vi "CMI ckd2 Set Divider Factor.vi"(8 "error in":errorcluster, 10 "division factor (1)":i32=1, 11 "session":T1) -> (0 "error out":errorcluster, 3 "session out":T1)   [LabVIEW 2020, in "AWG.lvlib"]
doc: "Sets division factor to main channel."
uses:
  AWG.lvlib
  CMI ckd2 Session.ctl
  CMI ckd2 Source Mode.ctl
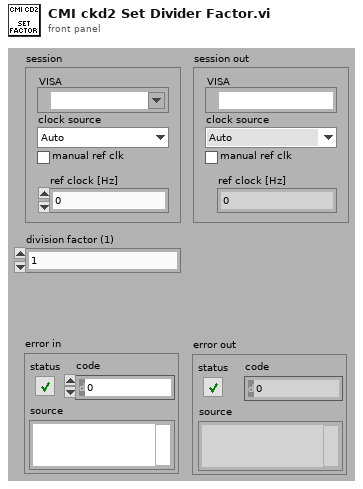
[diagram p1: front panel]
types:
  T1 = typedef "AWG.lvlib/CMI ckd2 Session.ctl" = cluster{"VISA":refnum<visa-resource-name>, "clock source":T2, "manual ref clk":bool, "ref clock [Hz]":dbl}
  T2 = typedef "AWG.lvlib/CMI ckd2 Source Mode.ctl" = enum16{"Auto", "LF clock", "HF clock", "Internal"}
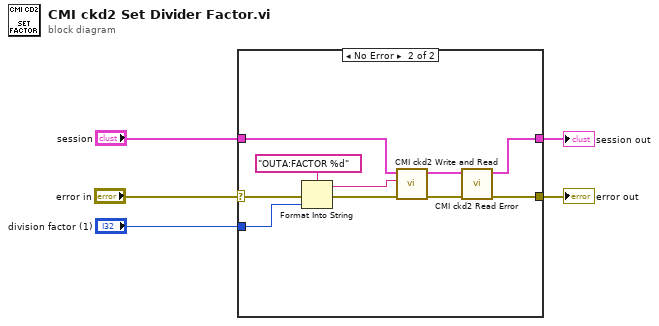
[diagram p0: block diagram]
diagram:
  n1 = case shown="No Error" "error in" {
    selector: "error in" -> [w6 w16]
    tunnel: [w7 w9] -> w3
    tunnel: [w6 w8] -> w5
    tunnel: "session" -> [w7 w17]
    tunnel: "division factor (1)" -> [_ w12]
    frame Error {
    }
    frame No Error {
      n2 = Format Into String(format string="OUTA:FACTOR %d", error in=w16, w12) -> (resulting string=w14:string, error out=w13:errorcluster)  [unwired: 1 in]
      n3 = call "CMI ckd2 Write and Read.vi"("error in"=w13, "command"=w14, "session"=w17) -> ("error out"=w11:errorcluster, "session out"=w10:T1)  [unwired: 6 in, 1 out]
      n4 = call "CMI ckd2 Read Error.vi"("error in"=w11, "session"=w10) -> ("error out"=w8:errorcluster, "session out"=w9:T1)  [unwired: 7 in, 1 out]
    }
  }
  "error out" <- w5
  "session out" <- w3
